vi "Linear Differential Equation Solving.vi"() -> ()   [LabVIEW 2023]
doc: "Demonstrates the use of the ODE Linear System Numeric VI to solve a system of linear differential equations."
uses:
  <vilib>/gmath/NI_Gmath.lvlib
panel:
  out "x(t)":cluster{"Times":dbl[], "X Values":dbl[]}[](graph)
  in  "Stop":bool
  in  "number of points":u32=256
  in  "end":dbl=7.0 format="%#.6g"
  in  "start":dbl format="%#.6g"
  out "error":i32
  in  "x0":dbl[](array[numeric])=[1.0, -2.0, 1.0, 2.0] format="%#.6g"
  in  "A":dbl[][](array[numeric])=[[-1.0, 1.0, -7.0, 0.0], [2.0, 2.0, 8.0, 3.0], [0.0, -1.0, -2.0, -1.0], [-1.0, -1.0, 0.0, -1.0]] format="%#.6g"
  # "Overview: Demonstrates the use of the ODE Linear System Numeric VI to solve a system of linear differential equations.\nRequirements: LabVIEW Full Development System\nInstructions:\n1. Run the VI.\n2. View the solution in the graph.\n3. Click Stop to stop the VI."
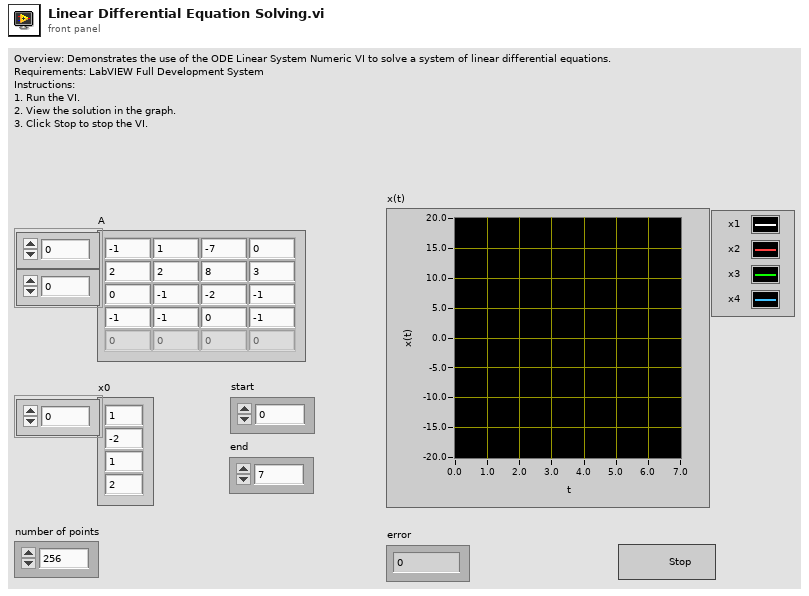
[diagram p1: front panel]
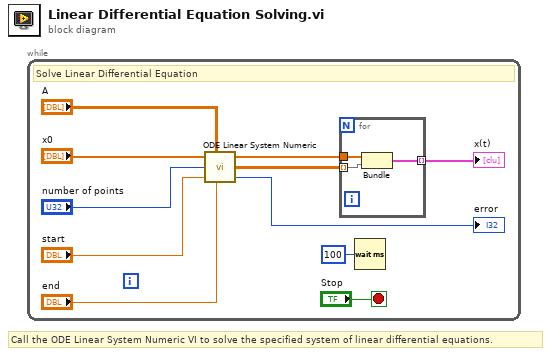
[diagram p0: block diagram]
diagram:
  # "Call the ODE Linear System Numeric VI to solve the specified system of linear differential equations."
  n1 = while {
    stop <- "Stop" stop-if-true
    # "Solve Linear Differential Equation"
    n2 = call <vilib>:"ODE Linear System Numeric.vi"("X0 (start value)"="x0", "A (matrix of coefficients)"="A", "number of points"="number of points", "time start"="start", "time end"="end") -> ("Times"=w6:dbl[], "X Values"=w5:dbl[][], "error"=→"error":i32)
    n3 = for {
      tunnel: w5 -> [w14] mode=indexing
      tunnel: w6 -> [w13]
      tunnel: [w12] -> w4 mode=indexing
      n4 = Bundle("Times"=w13, "X Values"=w14) -> (w12:cluster{"Times":dbl[], "X Values":dbl[]})  [unwired: 1 in]
    }
    "x(t)" <- w4
    n5 = Wait (ms)(milliseconds to wait=u32 100) -> ()  [unwired: 1 out]
  }
